vi "Guassian_2D.vi"(3 "output control":T1, 4 "data":T2, 5 "X":dbl[](array[numeric]), 6 "a":dbl[](array[numeric])) -> (0 "error out":errorcluster, 1 "f'(X,a)":dbl[][](array[numeric]), 2 "f(X,a)":dbl[](array[numeric]))   [LabVIEW 2016]
doc: "This template is the starting point for creating a model function to be passed to the Nonlinear Curve Fit.vi."
uses:
  <vilib>/gmath/NumericalOptimization/objective function data.ctl
  <vilib>/gmath/NumericalOptimization/LM_output select.ctl
  <vilib>/gmath/NI_Gmath.lvlib
panel:
  # "Amp\nXo\nYo\nWx\nWy\nOffset"
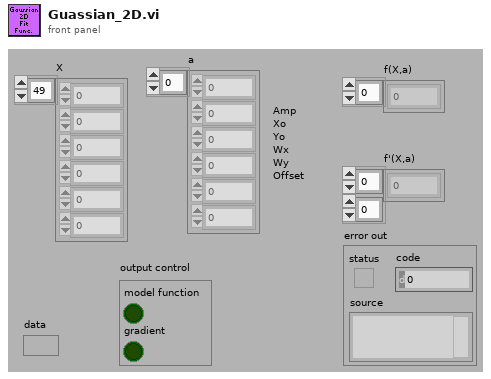
[diagram p1: front panel]
types:
  T1 = typedef "NI_Gmath.lvlib/LM_output select.ctl" = cluster{"model function":bool, "gradient":bool}
  T2 = typedef "NI_Gmath.lvlib/objective function data.ctl" = variant
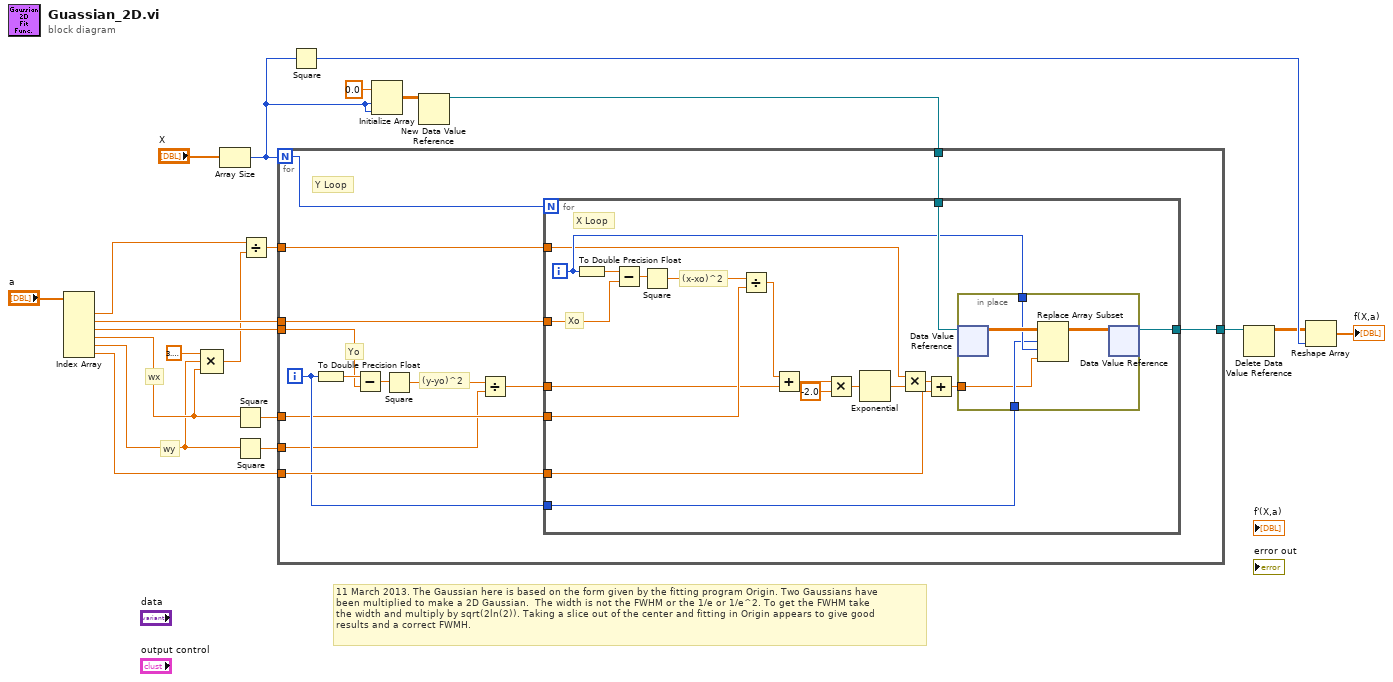
[diagram p0: block diagram]
diagram:
  # "11 March 2013. The Gaussian here is based on the form given by the fitting program Origin. Two Gaussians have\nbeen multiplied to make a 2D Gaussian.  The width is not the FWHM or the 1/e or 1/e^2. To get the FWHM take\nthe width and multiply by sqrt(2ln(2)). Taking a slice out of the center and fitting in Origin appears to give good\nresults and a correct FWMH."
  # "wy"
  # "wx"
  n1 = Index Array(array="a") -> (element #1=w4:dbl, element #2=w19:dbl, element #3=w18:dbl, element #4=w6:dbl, element #5=w5:dbl, element #6=w17:dbl)  [unwired: 6 in]
  n2 = Compound Arithmetic op=MULTIPLY(3.141592653589793, w5, w6) -> (w3:dbl)
  n3 = Array Size(array="X") -> (size(s)=w11:i32)
  n4 = Square(x=w6) -> (x^2=w9:dbl)
  n5 = Square(x=w5) -> (x^2=w8:dbl)
  n6 = Divide(x=w4, y=w3) -> (x/y=w2:dbl)
  n7 = Square(x=w11) -> (x^2=w10:i32)
  n8 = Initialize Array(0.0 ("element"), w11, w11) -> (w15:dbl[][])
  n9 = New Data Value Reference(data value=w15) -> (data value reference=w14:refnum<data-value>)  [unwired: 1 in, 1 out]
  n10 = for {
    N: w11 -> [w35]
    tunnel: w19 -> [w34]
    tunnel: w18 -> [w31]
    tunnel: w17 -> [w33]
    tunnel: w14 -> [w29]
    tunnel: [w27] -> w13
    tunnel: w9 -> [w26]
    tunnel: w8 -> [w24]
    tunnel: w2 -> [w22]
    i -> [w28]
    # "(y-yo)^2"
    # "Yo"
    # "Y Loop"
    n11 = To Double Precision Float(number=w28) -> (double precision float=w32:dbl)
    n12 = Subtract(x=w32, y=w31) -> (x-y=w30:dbl)
    n13 = Square(x=w30) -> (x^2=w25:dbl)
    n14 = Divide(x=w25, y=w24) -> (x/y=w23:dbl)
    n15 = for {
      N: w35 -> [_]
      tunnel: w34 -> [w53]
      tunnel: w33 -> [w51]
      tunnel: w29 -> [w50]
      tunnel: w28 -> [w48]
      tunnel: [w46] -> w27
      tunnel: w26 -> [w44]
      tunnel: w23 -> [w43]
      tunnel: w22 -> [w36]
      i -> [w49]
      # "Xo"
      # "(x-xo)^2"
      # "X Loop"
      n16 = To Double Precision Float(number=w49) -> (double precision float=w54:dbl)
      n17 = Subtract(x=w54, y=w53) -> (x-y=w52:dbl)
      n18 = Square(x=w52) -> (x^2=w45:dbl)
      n19 = Divide(x=w45, y=w44) -> (x/y=w42:dbl)
      n20 = Add(x=w42, y=w43) -> (x+y=w41:dbl)
      n21 = Multiply(x=w41, y=-2.0) -> (x*y=w39:dbl)
      n22 = Exponential(1:w39) -> (0:w38:dbl)
      n23 = Multiply(x=w36, y=w38) -> (x*y=w37:dbl)
      n24 = Add(x=w37, y=w51) -> (x+y=w47:dbl)
      n25 = in-place {
        in-place-border: w49 -> [w57]
        in-place-border: w48 -> [w56]
        in-place-border: w47 -> [w55]
        n26 = in-place-dvr #1(w50) -> (w59:dbl[][])  [unwired: 1 out]
        n27 = Replace Array Subset(array=w59, new element=w55, index (row)=w56, index (col)=w57) -> (w58:dbl[][])
        n28 = in-place-dvr #1(w58) -> (w46:refnum<data-value>)  [unwired: 1 out]
      }
    }
  }
  n29 = Delete Data Value Reference(data value reference=w13) -> (data value=w1:dbl[][])  [unwired: 1 in, 1 out]
  n30 = Reshape Array(w1, w10) -> (→"f(X,a)":dbl[])
